vi "Byte Value1.vi"(1 "Length":i32, 2 "Offset":u32, 3 "string":string) -> (0 "Value":i64)   [LabVIEW 2012]
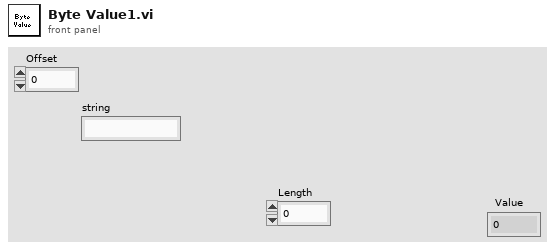
[diagram p1: front panel]
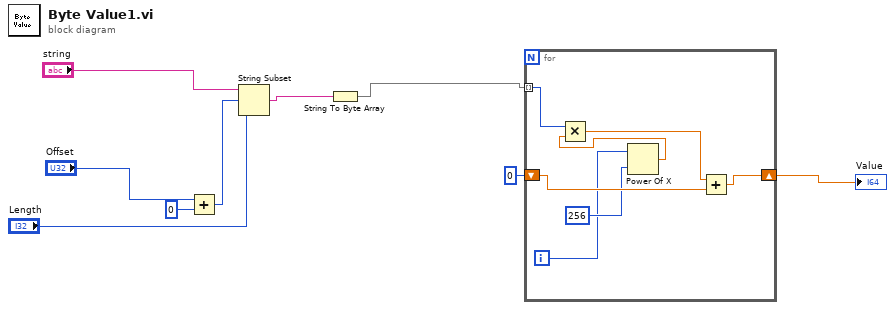
[diagram p0: block diagram]
diagram:
  n1 = Add(x="Offset", y=u32 0) -> (x+y=w7:u32)
  n2 = String Subset(string="string", offset (0)=w7, length (rest)="Length") -> (substring=w3:string)
  n3 = String To Byte Array(string=w3) -> (unsigned byte array=w6:u8[])
  n4 = for {
    tunnel: w6 -> [w16] mode=indexing
    shift-right: [w13] -> w4
    shift-left: 0 -> [w15]
    i -> [w10]
    n5 = Power Of X(1:256, 2:w10) -> (0:w12:dbl)
    n6 = Multiply(x=w16, y=w12) -> (x*y=w14:dbl)
    n7 = Add(x=w14, y=w15) -> (x+y=w13:dbl)
  }
  "Value" <- w4
